vi "Read PVF Param.vi"(8 "error in (no error)":errorcluster, 10 "Param Name":string, 11 "MatlabExperiment in":refnum<class "MatlabExperiment.lvclass">) -> (0 "error out":errorcluster, 2 "Param Value":string, 3 "MatlabExperiment out":refnum<class "MatlabExperiment.lvclass">)   [LabVIEW 2011, in "MatlabExperiment.lvclass"]
uses:
  MatlabExperiment.lvclass
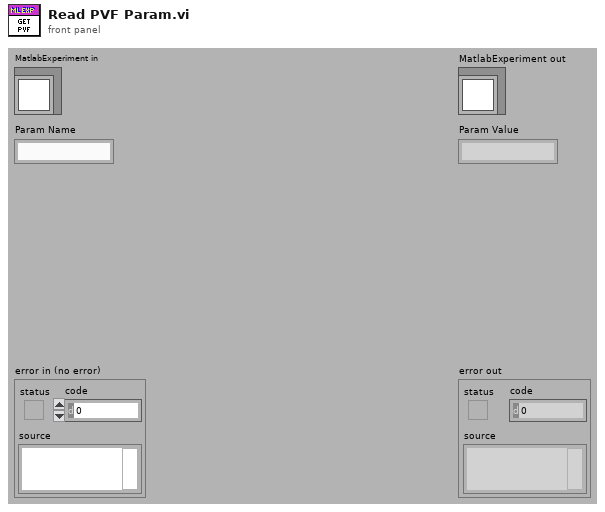
[diagram p1: front panel]
types:
  T1 = cluster{"Name":string, "Type":string, "value":string}[]
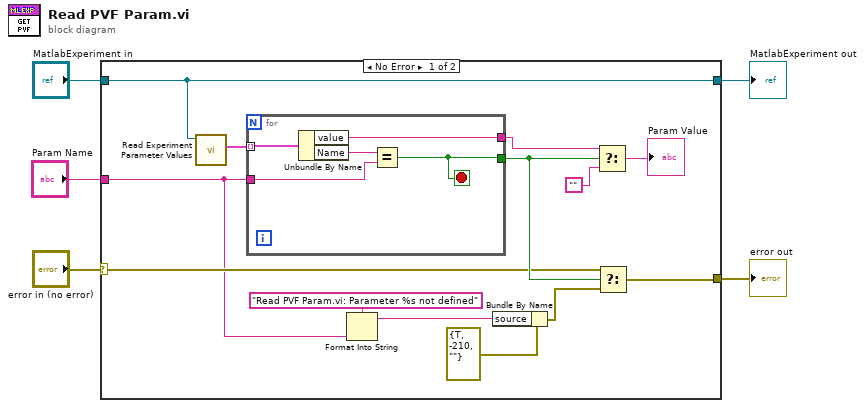
[diagram p0: block diagram]
diagram:
  n1 = case shown="No Error" "error in (no error)" {
    selector: "error in (no error)" -> [w12 w25]
    tunnel: [w11 w25] -> w4
    tunnel: [w18 w24] -> w2
    tunnel: "MatlabExperiment in" -> [w18 w24]
    tunnel: "Param Name" -> [w9 _]
    frame No Error {
      n2 = call-dynamic "Read Experiment Parameter Values.vi"("TrialBasedExperiment in"=w18) -> ("Experiment Parameter Values"=w17:T1)  [unwired: 8 in, 2 out]
      n3 = for {
        tunnel: w17 -> [w23] mode=indexing
        tunnel: w9 -> [w22]
        tunnel: [w20] -> w13
        tunnel: [w19] -> w16
        stop <- w20 stop-if-true
        n4 = Unbundle By Name(w23) -> ("value"=w19:string, "Name"=w21:string)
        n5 = Equal?(x=w21, y=w22) -> (x = y?=w20:bool)
      }
      n6 = Format Into String(format string="Read PVF Param.vi: Parameter %s not defined", w9) -> (resulting string=w8:string)  [unwired: 2 in, 1 out]
      n7 = Bundle By Name(cluster=errorcluster {"status"=TRUE, "code"=-210, "source"=""} ("f"), "source"=w8) -> (w6:errorcluster)
      n8 = Select(t=w16, s=w13, f="") -> (s? t:f=→"Param Value":string)
      n9 = Select(t=w12, s=w13, f=w6) -> (s? t:f=w11:errorcluster)
    }
    frame Error {
    }
  }
  "error out" <- w4
  "MatlabExperiment out" <- w2
